vi "MDML_publish_image.vi"(6 "connMeta":T1, 7 "Experiment ID 4":string, 8 "error in (no error)":errorcluster, 9 "String":string, 10 "DEVICE_ID":string, 11 "Path":path) -> (0 "error out":errorcluster)   [LabVIEW 2018]
uses:
  Downloads/mqtt_lv2013_201708181938/mqtt_lv2013/mqtt Folder/src/class/mqtt/mqttTypedef/mqttConnectionMeta.ctl
  Downloads/mqtt_lv2013_201708181938/mqtt_lv2013/mqtt Folder/src/class/mqtt/mqttTypedef/mqttQOSlevel.ctl
  image_message.ctl
  Downloads/mqtt_lv2013_201708181938/mqtt_lv2013/mqtt Folder/src/class/mqtt/mqtt.lvclass
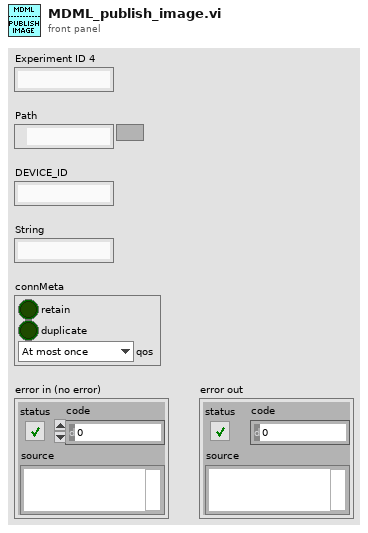
[diagram p1: front panel]
types:
  T1 = typedef "mqttConnectionMeta.ctl" = cluster{"retain":bool, "duplicate":bool, "qos":T2}
  T2 = typedef "mqttQOSlevel.ctl" = enum8{"At most once", "At least once", "Exactly once", "Reserved"}
  T3 = typedef "image_message.ctl" = cluster{"timestamp":string, "filename":string, "data":string, "data_type":string}
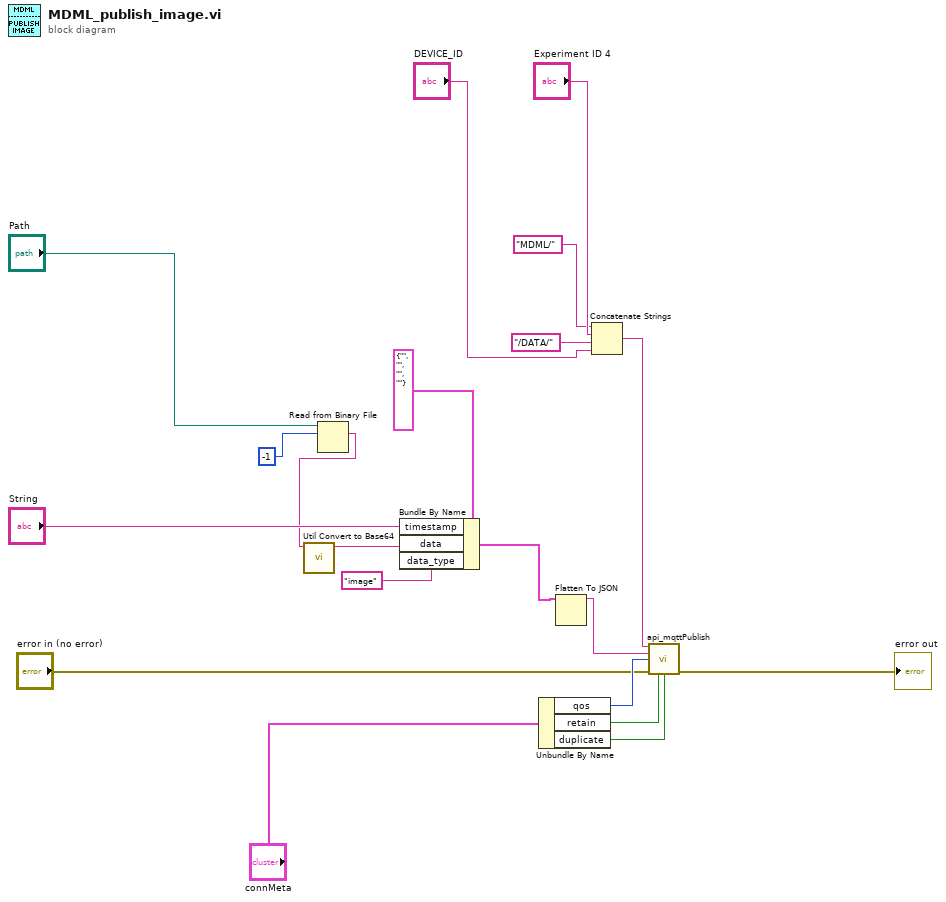
[diagram p0: block diagram]
diagram:
  n1 = Read from Binary File(10:-1, 11:"Path") -> (2:w14:string)  [unwired: 4 in, 3 out]
  n2 = call "Util Convert to Base64.vi"("String"=w14) -> ("Base64 String"=w15:string)  [unwired: 10 in]
  n3 = Bundle By Name(cluster=T3 {"timestamp"="", "filename"="", "data"="", "data_type"=""} ("input cluster"), "timestamp"="String", "data"=w15, "data_type"="image") -> (w12:T3)
  n4 = Unbundle By Name("connMeta") -> ("qos"=w5:T2, "retain"=w3:bool, "duplicate"=w4:bool)
  n5 = Flatten To JSON(anything=w12) -> (JSON string=w9:string)  [unwired: 2 in, 1 out]
  n6 = Concatenate Strings("MDML/", "Experiment ID 4", "/DATA/", "DEVICE_ID") -> (w8:string)
  n7 = call "api_mqttPublish.vi"("topic"=w8, "value"=w9, "QoS (At most once)"=w5, "error in (no error)"="error in (no error)", "retain(F)"=w3, "duplicate(F)"=w4) -> ("error out"=→"error out":errorcluster)  [unwired: 8 in, 1 out]
